vi "Get Configuration File Path.vi"(8 "error in (no error)":errorcluster caption="错误输入（无错误）") -> (0 "error out":errorcluster caption="错误输出", 3 "XML File Path":path caption="XML文件路径")   [LabVIEW 2013]
doc: "获取XML配置文件的路径。通过“应用程序目录”函数实现。关于“应用程序目录”函数如何计算路径的更多信息，可右键单击函数并选择“帮助”。"
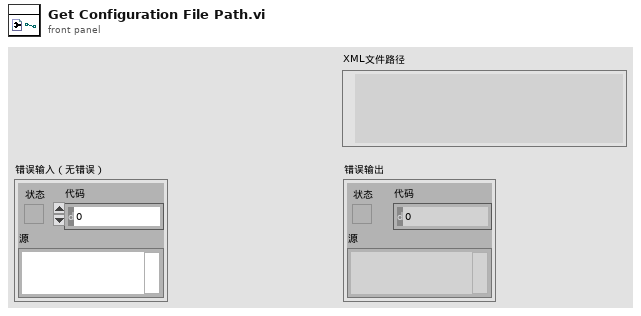
[diagram p1: front panel]
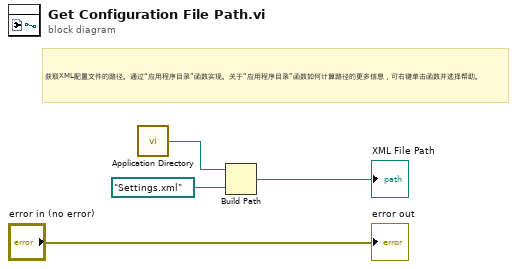
[diagram p0: block diagram]
diagram:
  # "获取XML配置文件的路径。通过“应用程序目录”函数实现。关于“应用程序目录”函数如何计算路径的更多信息，可右键单击函数并选择帮助。"
  n1 = call <vilib>:"Application Directory.vi"() -> ("Application Directory"=w1:path)
  n2 = Build Path(base path=w1, name or relative path=path "Settings.xml" ("string")) -> (appended path=→"XML File Path":path)
  "error out" <- "error in (no error)"
